vi "Pixel 1.2.vi"() -> ()   [LabVIEW 2018]
panel:
  in  "VISA Refnum in":refnum<visa-resource-name>="ASRL5::INSTR"
  in  "Start Game/Robots turn":bool
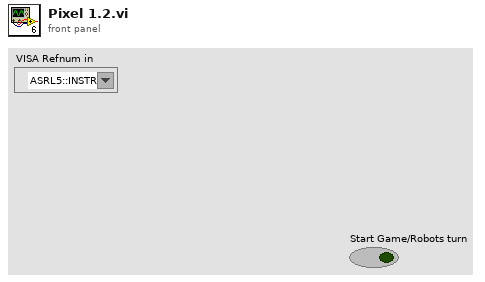
[diagram p1: front panel]
types:
  T1 = enum16{"Child's Turn", "Robot's Turn", "Waiting State", "Game Over"}
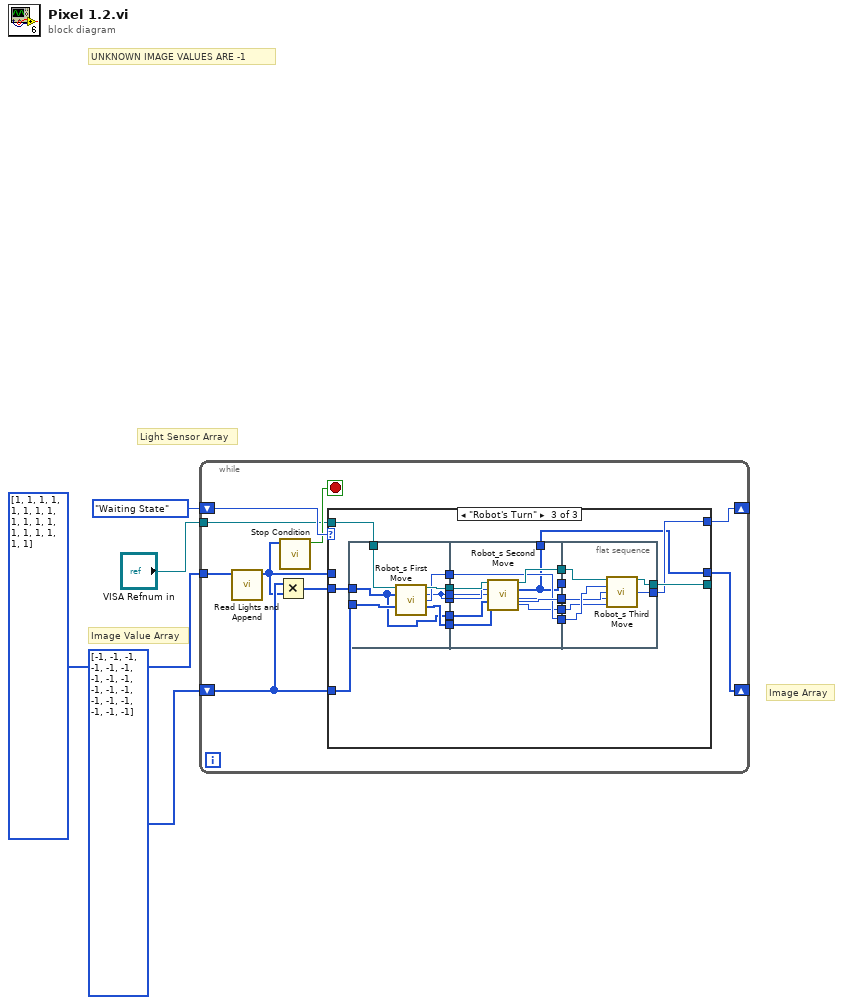
[diagram p0: block diagram]
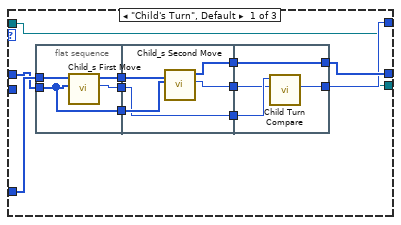
[diagram p2: hidden frame]
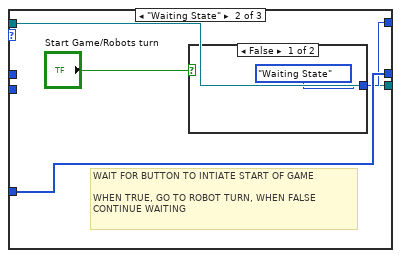
[diagram p3: hidden frame]
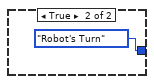
[diagram p4: hidden frame]
diagram:
  # "Image Array"
  # "UNKNOWN IMAGE VALUES ARE -1"
  # "Light Sensor Array"
  # "Image Value Array"
  n1 = while {
    shift-right: [w6] -> _
    shift-left: T1."Waiting State" -> [w13]
    shift-right: [w10] -> _
    shift-left: i32[] [-1, -1, -1, -1, -1, -1, -1, -1, -1, -1, -1, -1, -1, -1, -1, -1, -1, -1] ("Array") -> [w8]
    tunnel: i32[] [1, 1, 1, 1, 1, 1, 1, 1, 1, 1, 1, 1, 1, 1, 1, 1, 1, 1] ("Array") -> [w9]
    tunnel: "VISA Refnum in" -> [w5]
    stop <- w12 stop-if-true
    n2 = call "Read Lights and Append.vi"("Input (Old) Light Sensor Array"=w9) -> ("Output Light Sensor Array"=w7:i32[])  [unwired: 7 in]
    n3 = Multiply(x=w8, y=w7) -> (x*y=w11:i32[])
    n4 = call "Stop Condition.vi"("Light Sensor Array"=w7) -> ("element"=w12:bool)  [unwired: 10 in]
    n5 = case shown="\"Robot's Turn\"" w13 {
      tunnel: w11 -> [_ _ w61]
      tunnel: [w19 w40 w44] -> w10
      tunnel: [w14 w38 w58] -> _
      tunnel: w8 -> [w24 w40 w57]
      tunnel: w7 -> [w23 _ _]
      tunnel: [w15 w39 w46] -> w6
      tunnel: w5 -> [w14 w38 w45]
      frame "Child's Turn", Default {
        n6 = flat-sequence {
          tunnel: w24 -> [w28]
          tunnel: w23 -> [w26]
          tunnel: [w27] -> w22
          tunnel: [w26] -> w21
          tunnel: [w25] -> w18
          tunnel: w22 -> [w33]
          tunnel: w21 -> [w32]
          tunnel: [w31] -> w20
          tunnel: w18 -> [w30]
          tunnel: [w30] -> w17
          tunnel: [w29] -> w16
          tunnel: [w37] -> w19
          tunnel: w20 -> [w37]
          tunnel: w17 -> [w36]
          tunnel: w16 -> [w35]
          tunnel: [w34] -> w15
          frame #0 {
            n7 = call "Child_s First Move.vi"("Old Light Sensor Array"=w26, "Current Image Array"=w28) -> ("Image Value From First Turn"=w25:i32, "Output Image Array"=w27:i32[])  [unwired: 8 in]
          }
          frame #1 {
            n8 = call "Child_s Second Move.vi"("Old Light Sensor Array"=w32, "Current Image Array"=w33) -> ("Image Value From Second Turn"=w29:i32, "Output Image Array"=w31:i32[])  [unwired: 8 in]
          }
          frame #2 {
            n9 = call "Child Turn Compare.vi"("Image Value from Second Move"=w35, "Image value from First Move"=w36) -> ("Next Move"=w34:T1)  [unwired: 9 in]
          }
        }
      }
      frame "Waiting State" {
        # "WAIT FOR BUTTON TO INTIATE START OF GAME\n\nWHEN TRUE, GO TO ROBOT TURN, WHEN FALSE \nCONTINUE WAITING"
        n10 = case shown="False" "Start Game/Robots turn" {
          tunnel: [T1."Waiting State" T1."Robot's Turn"] -> w39
          frame False {
          }
          frame True {
          }
        }
      }
      frame "Robot's Turn" {
        n11 = flat-sequence {
          tunnel: w61 -> [w65]
          tunnel: [w68] -> w60
          tunnel: [w67] -> w59
          tunnel: w57 -> [w66]
          tunnel: [w63] -> w56
          tunnel: [w65] -> w55
          tunnel: [w64] -> w50
          tunnel: [w63] -> w47
          tunnel: w45 -> [w62]
          tunnel: w60 -> [w78]
          tunnel: w59 -> [w75]
          tunnel: w56 -> [w77]
          tunnel: w55 -> [w76]
          tunnel: [w74] -> w54
          tunnel: [w69] -> w53
          tunnel: [w73] -> w52
          tunnel: [w72] -> w51
          tunnel: w50 -> [w72]
          tunnel: [w71] -> w49
          tunnel: [w70] -> w48
          tunnel: w47 -> [w70]
          tunnel: [w69] -> w44
          tunnel: [w85] -> w58
          tunnel: w54 -> [w84]
          tunnel: w53 -> [_]
          tunnel: w52 -> [w82]
          tunnel: w51 -> [w83]
          tunnel: w49 -> [w81]
          tunnel: w48 -> [w80]
          tunnel: [w79] -> w46
          frame #0 {
            n12 = call "Robot_s First Move.vi"("VISA Refnum in"=w62, "In Play Array"=w65, "Current Image Array 2"=w66) -> ("VISA Refnum out"=w68:refnum<visa-resource-name>, "Index From First Move"=w63:i32, "Image Value from First Turn"=w64:i32, "Output Image Array"=w67:i32[])  [unwired: 8 in, 1 out]
          }
          frame #1 {
            n13 = call "Robot_s Second Move.vi"("VISA Refnum in"=w78, "Index from First Move"=w77, "In Play Array"=w76, "Current Image Array"=w75) -> ("VISA Refnum out"=w74:refnum<visa-resource-name>, "Output Image Array"=w69:i32[], "Image Value from Second Turn"=w73:i32, "Index From Second Move"=w71:i32)  [unwired: 7 in, 1 out]
          }
          frame #2 {
            n14 = call "Robot_s Third Move.vi"("Machine In"=w84, "Image Value From First Turn"=w83, "Image  value From Second Turn"=w82, "Index From First Move"=w80, "Index From Second Move"=w81) -> ("Machine Out"=w85:refnum<visa-resource-name>, "Next Move"=w79:enum16{"Child's Turn", "Robot's Turn"})  [unwired: 8 in, 1 out]
          }
        }
      }
    }
  }
